vi "ImageDisplay.vi"(7 "Frame":i32(slide) min=0 max=3507 step=1 scale=0.0..3507.0, 9 "Path":path, 10 "JPG or AVI":bool) -> (1 "Number of frames":dbl, 2 "Frames":u32[](array[numeric]), 3 "Image":T1(plugin-control))   [LabVIEW 2015]
uses:
  <vilib>/vision/NI_Vision_Development_Module.lvlib
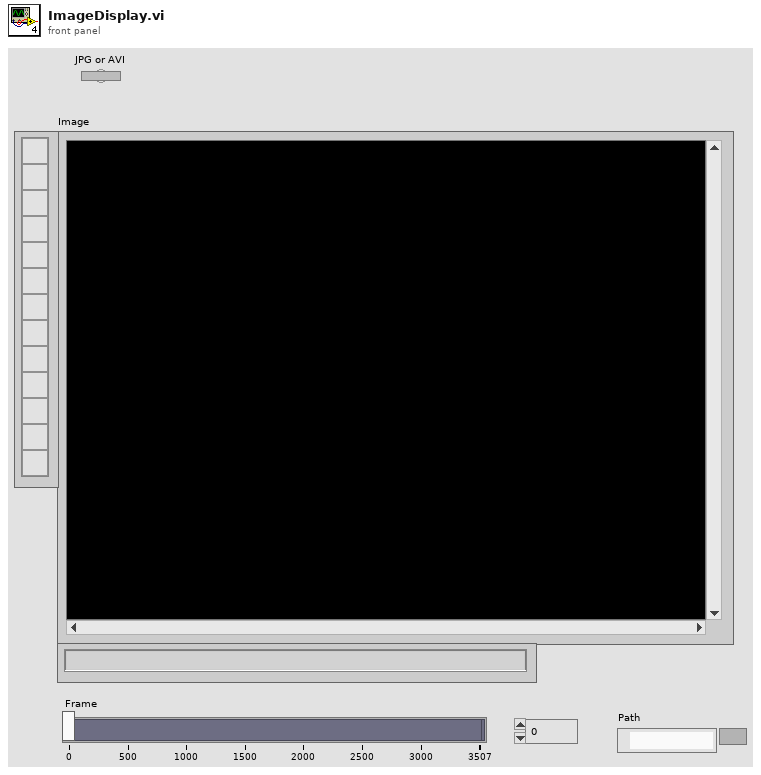
[diagram p1: front panel]
types:
  T1 = typedef "IMAQ Image.ctl" = refnum<image>
  T2 = typedef "Image Type" = u32
  T3 = typedef "IMAQ AVI2 Refnum.ctl" = refnum<k20>
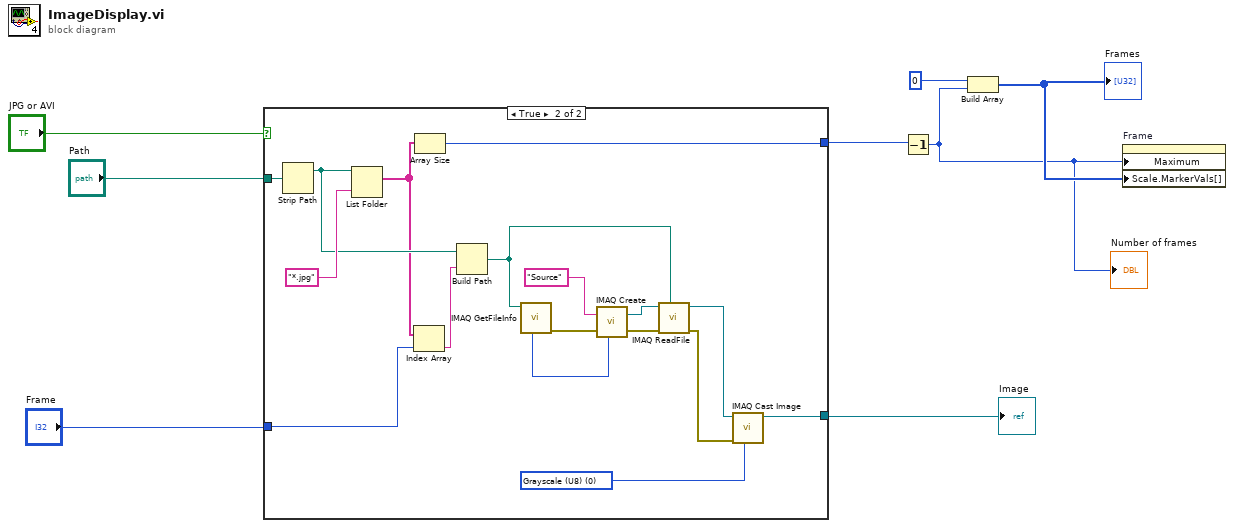
[diagram p0: block diagram]
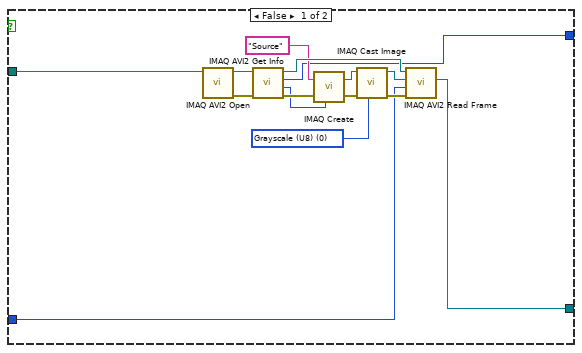
[diagram p2: hidden frame]
diagram:
  n1 = case shown="True" "JPG or AVI" {
    tunnel: "Path" -> [w23 w31]
    tunnel: [w13 w33] -> w6
    tunnel: [w9 w25] -> w4
    tunnel: "Frame" -> [w10 w26]
    frame False {
      w12 = T2 0 items=["Grayscale (U8)", "Grayscale (I16)", "Grayscale (SGL)", "Complex (CSG)", "RGB (U32)", "HSL (U32)", "RGB (U64)", "Grayscale (U16)"] ("Image Type")
      n2 = call "IMAQ AVI2 Open"("AVI File Path"=w23) -> ("error out"=w22:errorcluster, "AVI Refnum"=w21:T3)  [unwired: 9 in]
      n3 = call "IMAQ AVI2 Get Info"("error in (no error)"=w22, "AVI Refnum"=w21) -> ("error out"=w17:errorcluster, "Image Type"=w11:T2, "Number of Frames"=w9:u32, "AVI Refnum (duplicate)"=w20:T3)  [unwired: 5 in, 1 out]
      n4 = call "IMAQ Create"("Image Name"="Source", "Image Type"=w11, "error in (no error)"=w17) -> ("New Image"=w19:T1, "error out"=w18:errorcluster)  [unwired: 2 in]
      n5 = call "IMAQ Cast Image"("Image Type"=w12, "error in (no error)"=w18, "Image Src"=w19) -> ("error out"=w14:errorcluster, "Image Dst Out"=w15:T1)  [unwired: 7 in]
      n6 = call "IMAQ AVI2 Read Frame"("error in (no error)"=w14, "Frame Number"=w10, "Image"=w15, "AVI Refnum"=w20) -> ("Image Out"=w13:T1)  [unwired: 5 in, 2 out]
    }
    frame True {
      w32 = T2 0 items=["Grayscale (U8)", "Grayscale (I16)", "Grayscale (SGL)", "Complex (CSG)", "RGB (U32)", "HSL (U32)", "RGB (U64)", "Grayscale (U16)"] ("Image Type")
      n7 = Strip Path(path=w31) -> (stripped path=w28:path)  [unwired: 1 out]
      n8 = List Folder(path=w28, pattern="*.jpg") -> (filenames=w24:string[])  [unwired: 2 in, 3 out]
      n9 = Index Array(array=w24, index=w26) -> (element=w29:string)
      n10 = Array Size(array=w24) -> (size(s)=w25:i32)
      n11 = Build Path(base path=w28, name or relative path=w29) -> (appended path=w27:path)
      n12 = call "IMAQ GetFileInfo"("File Path"=w27) -> ("error out"=w37:errorcluster, "Image Type"=w36:T2)  [unwired: 4 in, 5 out]
      n13 = call "IMAQ Create"("Image Name"="Source", "Image Type"=w36, "error in (no error)"=w37) -> ("New Image"=w40:T1, "error out"=w39:errorcluster)  [unwired: 2 in]
      n14 = call "IMAQ ReadFile"("File Path"=w27, "error in (no error)"=w39, "Image"=w40) -> ("error out"=w35:errorcluster, "Image Out"=w34:T1)  [unwired: 4 in, 3 out]
      n15 = call "IMAQ Cast Image"("Image Type"=w32, "error in (no error)"=w35, "Image Src"=w34) -> ("Image Dst Out"=w33:T1)  [unwired: 7 in, 1 out]
    }
  }
  "Image" <- w6
  n16 = Decrement(x=w4) -> (x-1=w1:u32)
  "Number of frames" <- w1
  n17 = Build Array(0, w1) -> (w2:u32[])
  "Frames" <- w2
  n18 = property on="Frame" class="Slide (strict)"("Maximum"=w1, "Scale.MarkerVals[]"=w2) -> ()  [unwired: 2 in, 2 out]
